vi "SDG60LoadPolarity.vi"(1 "Channel (1: Channel1)":u16(ring)=1 items=["Channel1"=1, "Channel2"=2], 2 "Impedance (50.0 Ohms)":dbl=50.0 format="%#_15g", 4 "Polarity (0: Normal)":u16(ring) items=["Normal", "Inverted"]) -> ()   [LabVIEW 2022 SP3]
doc: "Configures the output impedance and source impedance for the channel you specify."
uses:
  <vilib>/addons/zeromq/socket_type.ctl
  <vilib>/addons/zeromq/zmq_context.lvclass
  <vilib>/addons/zeromq/zmq_socket.lvclass
  <vilib>/addons/zeromq/zeromq.lvlib
panel:
  out "resulting string":string
  out "Python response":string
  # "50..100K, or HiZ if larger"
  # "Changing impedance changes the\nset amplitude to maintain the same output amplitued"
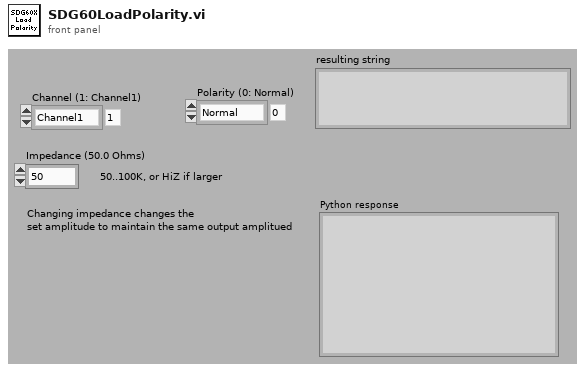
[diagram p1: front panel]
types:
  T1 = typedef "zeromq.lvlib/socket_type.ctl" = enum8{"ZMQ_PAIR", "ZMQ_PUB", "ZMQ_SUB", "ZMQ_REQ", "ZMQ_REP", "ZMQ_DEALER", "ZMQ_ROUTER", "ZMQ_PULL", "ZMQ_PUSH", "ZMQ_XPUB", "ZMQ_XSUB", "ZMQ_STREAM", "ZMQ_SERVER", "ZMQ_CLIENT", "ZMQ_RADIO", "ZMQ_DISH", "ZMQ_GATHER", "ZMQ_SCATTER", "ZMQ_DGRAM"}
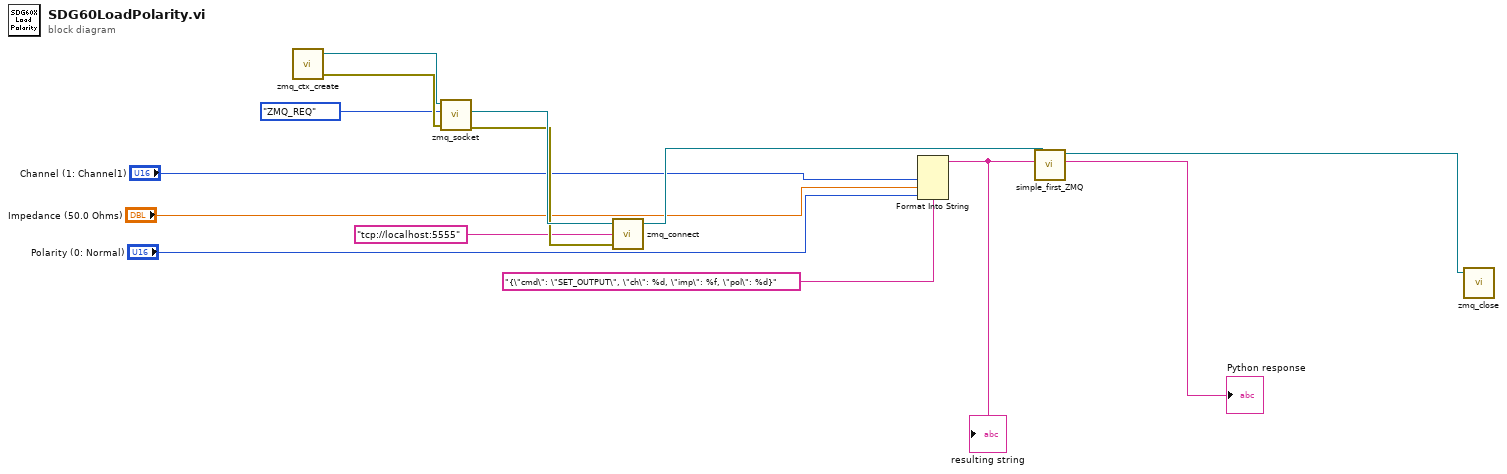
[diagram p0: block diagram]
diagram:
  n1 = call <vilib>:"zmq_ctx_create.vi"() -> ("error out"=w12:errorcluster, "context out"=w14:refnum<class "zmq_context.lvclass">)  [unwired: 4 in]
  n2 = call <vilib>:"zmq_socket.vi"("error in"=w12, "socket type"=socket_type."ZMQ_REQ", "context in"=w14) -> ("error out"=w11:errorcluster, "socket out"=w13:refnum<class "zmq_socket.lvclass">)  [unwired: 2 in, 1 out]
  n3 = call <vilib>:"zmq_connect.vi"("error in"=w11, "endpoint"="tcp://localhost:5555", "socket in"=w13) -> ("socket out"=w8:refnum<class "zmq_socket.lvclass">)  [unwired: 1 in, 1 out]
  n4 = Format Into String(format string="{\"cmd\": \"SET_OUTPUT\", \"ch\": %d, \"imp\": %f, \"pol\": %d}", "Channel (1: Channel1)", "Impedance (50.0 Ohms)", "Polarity (0: Normal)") -> (resulting string=w7:string)  [unwired: 2 in, 1 out]
  "resulting string" <- w7
  n5 = call "simple_first_ZMQ.vi"("Raw command"=w7, "ZMQ socket in"=w8) -> ("Python response"=→"Python response":string, "ZMQ socket out"=w6:refnum<class "zmq_socket.lvclass">)  [unwired: 4 in]
  n6 = call <vilib>:"zmq_close.vi"("socket"=w6) -> ()  [unwired: 4 in, 1 out]
